vi "Read UDP Resource.vi"(8 "error in (no error)":errorcluster, 11 "LiDAR in":refnum<class "Telnet V2.lvclass">) -> (0 "error out":errorcluster, 2 "UDP":T1, 3 "LiDAR out":refnum<class "Telnet V2.lvclass">)   [LabVIEW 2018]
uses:
  Telnet V2.lvclass
  C:/AME Test Engineering/LabVIEW/PPLs/LiDAR/Parent/LiDAR.lvlibp/LiDAR.lvclass
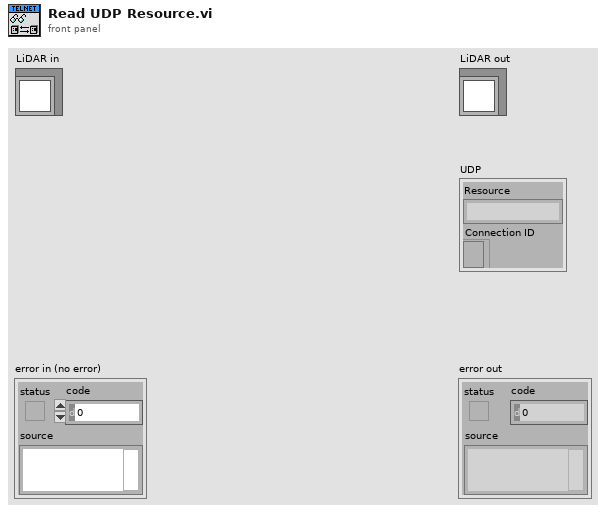
[diagram p1: front panel]
types:
  T1 = cluster{"Resource":string, "Connection ID":refnum<k5>}
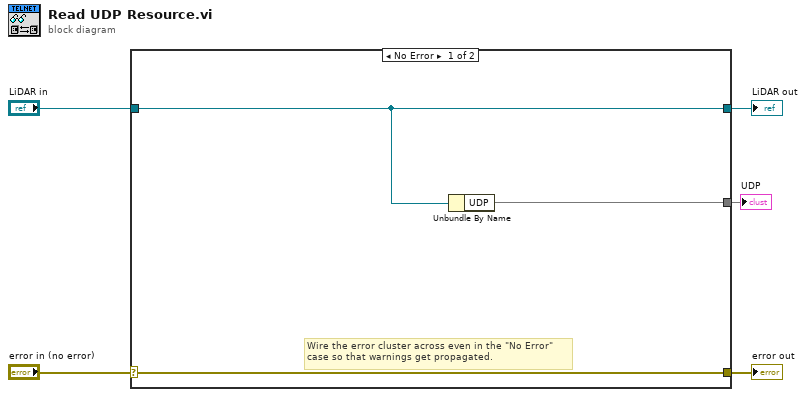
[diagram p0: block diagram]
diagram:
  n1 = case shown="No Error" "error in (no error)" {
    selector: "error in (no error)" -> [w8 w10]
    tunnel: [w8 w10] -> w4
    tunnel: [w7 w9] -> w2
    tunnel: "LiDAR in" -> [w7 w9]
    tunnel: [w6 _] -> w1
    frame No Error {
      # "Wire the error cluster across even in the \"No Error\"\ncase so that warnings get propagated."
      n2 = Unbundle By Name(w7) -> ("UDP"=w6)
    }
    frame Error {
    }
  }
  "error out" <- w4
  "LiDAR out" <- w2
  "UDP" <- w1
